vi "Color Match.vi"() -> ()   [LabVIEW 2019]
uses:
  Framework/Robot Global Data.vi
  <vilib>/regexp/Match Regular Expression.xnode
panel:
  out "Color to Match":string
  out "Correct Color":bool
  out "Matched Color Name":string
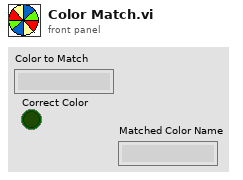
[diagram p1: front panel]
types:
  T1 = typedef "Color Sensor V3 DevRef.ctl" = cluster{"I2CDevRef":T2}
  T2 = typedef "WPI_I2CDevRef.ctl" = cluster{"DevStatus":errorcluster, "Device Address":u8, "Handle":i32, "I2C Bus":T3}
  T3 = typedef "i2c_bus.ctl" = enum16{"I2C On-Board", "I2C MXP", "Invalid"}
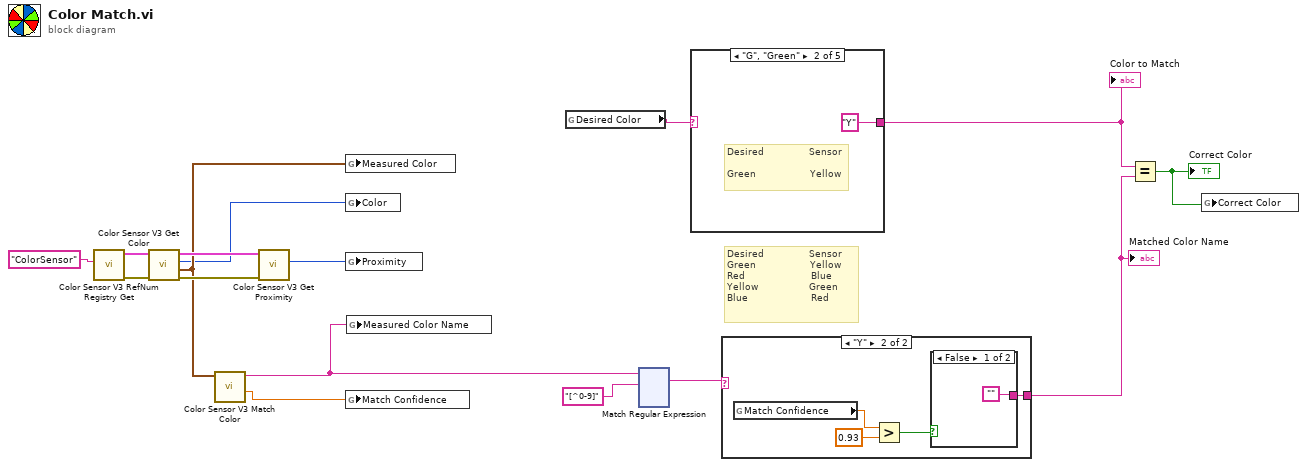
[diagram p0: block diagram]
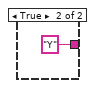
[diagram p3: hidden frame]
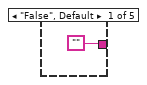
[diagram p4: hidden frame]
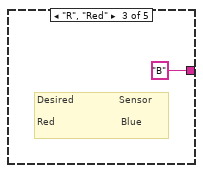
[diagram p5: hidden frame]
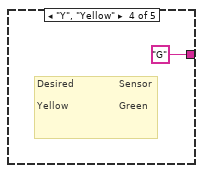
[diagram p6: hidden frame]
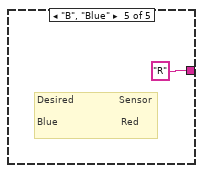
[diagram p7: hidden frame]
diagram:
  # "Desired               Sensor\nGreen                  Yellow\nRed                      Blue       \nYellow                 Green\nBlue                     Red"
  n1 = call <vilib>:"Color Sensor V3 RefNum Registry Get.vi"("refnum name"="ColorSensor") -> ("error out"=w14:errorcluster, "ColorSensorDevRef"=w13:T1)  [unwired: 9 in]
  n2 = call <vilib>:"Color Sensor V3 Get Color.vi"("error in (no error)"=w14, "ColorSensorDevRef"=w13) -> ("error out"=w16:errorcluster, "Normalized Color"=w11:cluster{"R":dbl, "G":dbl, "B":dbl}, "Color"=w10:u32, "ColorSensorDevRef out"=w15:T1)  [unwired: 6 in]
  n3 = call <vilib>:"Color Sensor V3 Match Color.vi"("Measured Color"=w11) -> ("Confidence"=w8:dbl, "Matched Color Name"=w1:string)  [unwired: 8 in, 1 out]
  n4 = call <vilib>:"Color Sensor V3 Get Proximity.vi"("error in (no error)"=w16, "ColorSensorDevRef"=w15) -> ("Proximity"=w9:u16)  [unwired: 7 in, 2 out]
  n5 = global write "Robot Global Data.vi" "Measured Color"(w11) -> ()
  n6 = global write "Robot Global Data.vi" "Color"(w10) -> ()
  n7 = global write "Robot Global Data.vi" "Proximity"(w9) -> ()
  n8 = global write "Robot Global Data.vi" "Match Confidence"(w8) -> ()
  n9 = global write "Robot Global Data.vi" "Measured Color Name"(w1) -> ()
  n10 = global read "Robot Global Data.vi" "Desired Color"() -> (w2:string)
  n11 = xnode "Match Regular Expression"("input string"=w1, "regular expression"="[^0-9]") -> ("whole match"=w5:string)  [unwired: 4 in, 4 out]
  n12 = case shown="\"G\", \"Green\"" w2 {
    tunnel: ["" "Y" "B" "G" "R"] -> w3
    frame "False", Default {
    }
    frame "G", "Green" {
      # "Desired               Sensor\n\nGreen                  Yellow"
    }
    frame "R", "Red" {
      # "Desired               Sensor\n\nRed                      Blue"
    }
    frame "Y", "Yellow" {
      # "Desired               Sensor\n\nYellow                 Green"
    }
    frame "B", "Blue" {
      # "Desired               Sensor\n\nBlue                     Red"
    }
  }
  "Color to Match" <- w3
  n13 = case shown="\"Y\"" w5 {
    selector: w5 -> [w22 _]
    tunnel: [w22 w23] -> w6
    frame Default {
    }
    frame "Y" {
      n14 = global read "Robot Global Data.vi" "Match Confidence"() -> (w26:dbl)
      n15 = Greater?(x=w26, y=0.93) -> (0:w24:bool)
      n16 = case shown="False" w24 {
        tunnel: ["" "Y"] -> w23
        frame False {
        }
        frame True {
        }
      }
    }
  }
  "Matched Color Name" <- w6
  n17 = Equal?(x=w3, y=w6) -> (x = y?=w7:bool)
  "Correct Color" <- w7
  n18 = global write "Robot Global Data.vi" "Correct Color"(w7) -> ()
